vi "Check Grape Time.vi"(8 "error in (no error)":errorcluster, 11 "Grape in":refnum<class "Grape.lvclass">) -> (0 "error out":errorcluster, 3 "Grape out":refnum<class "Grape.lvclass">)   [LabVIEW 2021, in "Grape.lvclass"]
uses:
  Grape.lvclass
  C:/Users/poche/Programs/LabVIEW/imposible snake/GameEl_class/GameEl.lvclass
  Grape.lvclass/Grape.ctl
  GameEl_class/GameEl.lvclass/GameEl.ctl
  GameEl_class/GameEl.lvclass
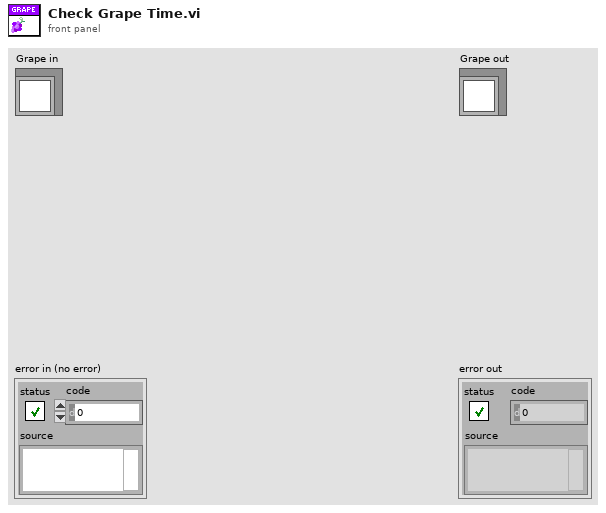
[diagram p1: front panel]
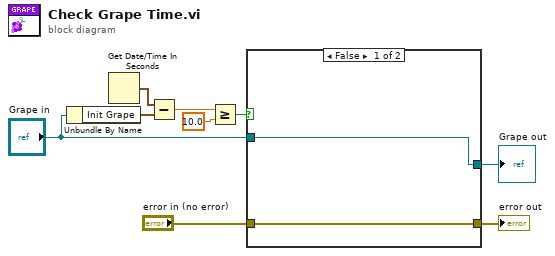
[diagram p0: block diagram]
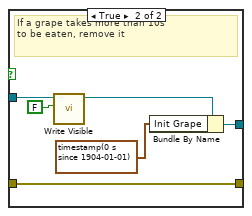
[diagram p2: hidden frame]
diagram:
  n1 = Unbundle By Name("Grape in") -> ("Init Grape"=w8:timestamp)
  n2 = Get Date/Time In Seconds() -> (seconds since 1Jan1904=w9:timestamp)
  n3 = Subtract(x=w9, y=w8) -> (x-y=w7:dbl)
  n4 = Greater Or Equal?(x=w7, y=10.0) -> (x >= y?=w5:bool)
  n5 = case shown="False" w5 {
    tunnel: "Grape in" -> [w11 w17]
    tunnel: [w11 w16] -> w3
    tunnel: "error in (no error)" -> [w10 w14]
    tunnel: [w10 w14] -> w1
    frame False {
    }
    frame True {
      # "If a grape takes more than 10s\nto be eaten, remove it"
      n6 = call "Write Visible.vi"("Visible"=FALSE, "GameEl in"=w17) -> ("GameEl out"=w13:refnum<class "Grape.lvclass">)  [unwired: 8 in, 1 out]
      n7 = Bundle By Name(cluster=w13, "Init Grape"=timestamp(0 s since 1904-01-01) ("Init Shield")) -> (w16:refnum<class "Grape.lvclass">)
    }
  }
  "error out" <- w1
  "Grape out" <- w3
